vi "DAQ PID.vi"() -> ()   [LabVIEW 2024]
uses:
  <vilib>/addons/control/pid/pid.llb/PID (DBL).vi
  <vilib>/addons/control/pid/NI_PID_pid.lvlib
panel:
  out "2":bool
  out "1":bool
  out "ANG ACT":dbl
  out "error":dbl
  in  "stop":bool
  out "DERECHA":dbl
  out "IZQUIERDA":dbl
  out "P-A":dbl
  out "P-B":dbl
  out "DER":bool
  out "IZQ":bool
  out "PULSOS TOTALES":dbl
  in  "ANGULO":i16(knob) scale=-180.0..180.0
  in  "PID gains":T1 {"derivative time (Td, min)" format="%.3f"; "integral time (Ti, min)" format="%.3f"; "proportional gain (Kc)" format="%.3f"}
  out "ERROR":dbl(graph)
  out "PWM":dynamicdata(graph)
  out "SALIDA PID":dbl
  in  "output range":cluster{"output high":dbl, "output low":dbl} {"output low" format="%.2f"; "output high" format="%.2f"}
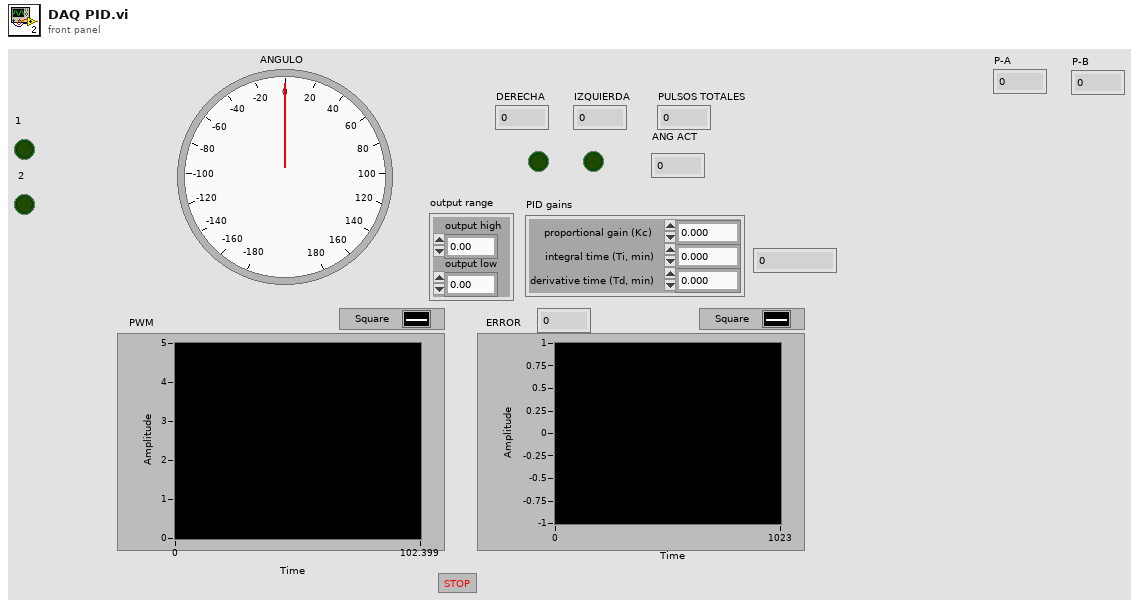
[diagram p1: front panel]
types:
  T1 = cluster{"proportional gain (Kc)":dbl, "integral time (Ti, min)":dbl, "derivative time (Td, min)":dbl}
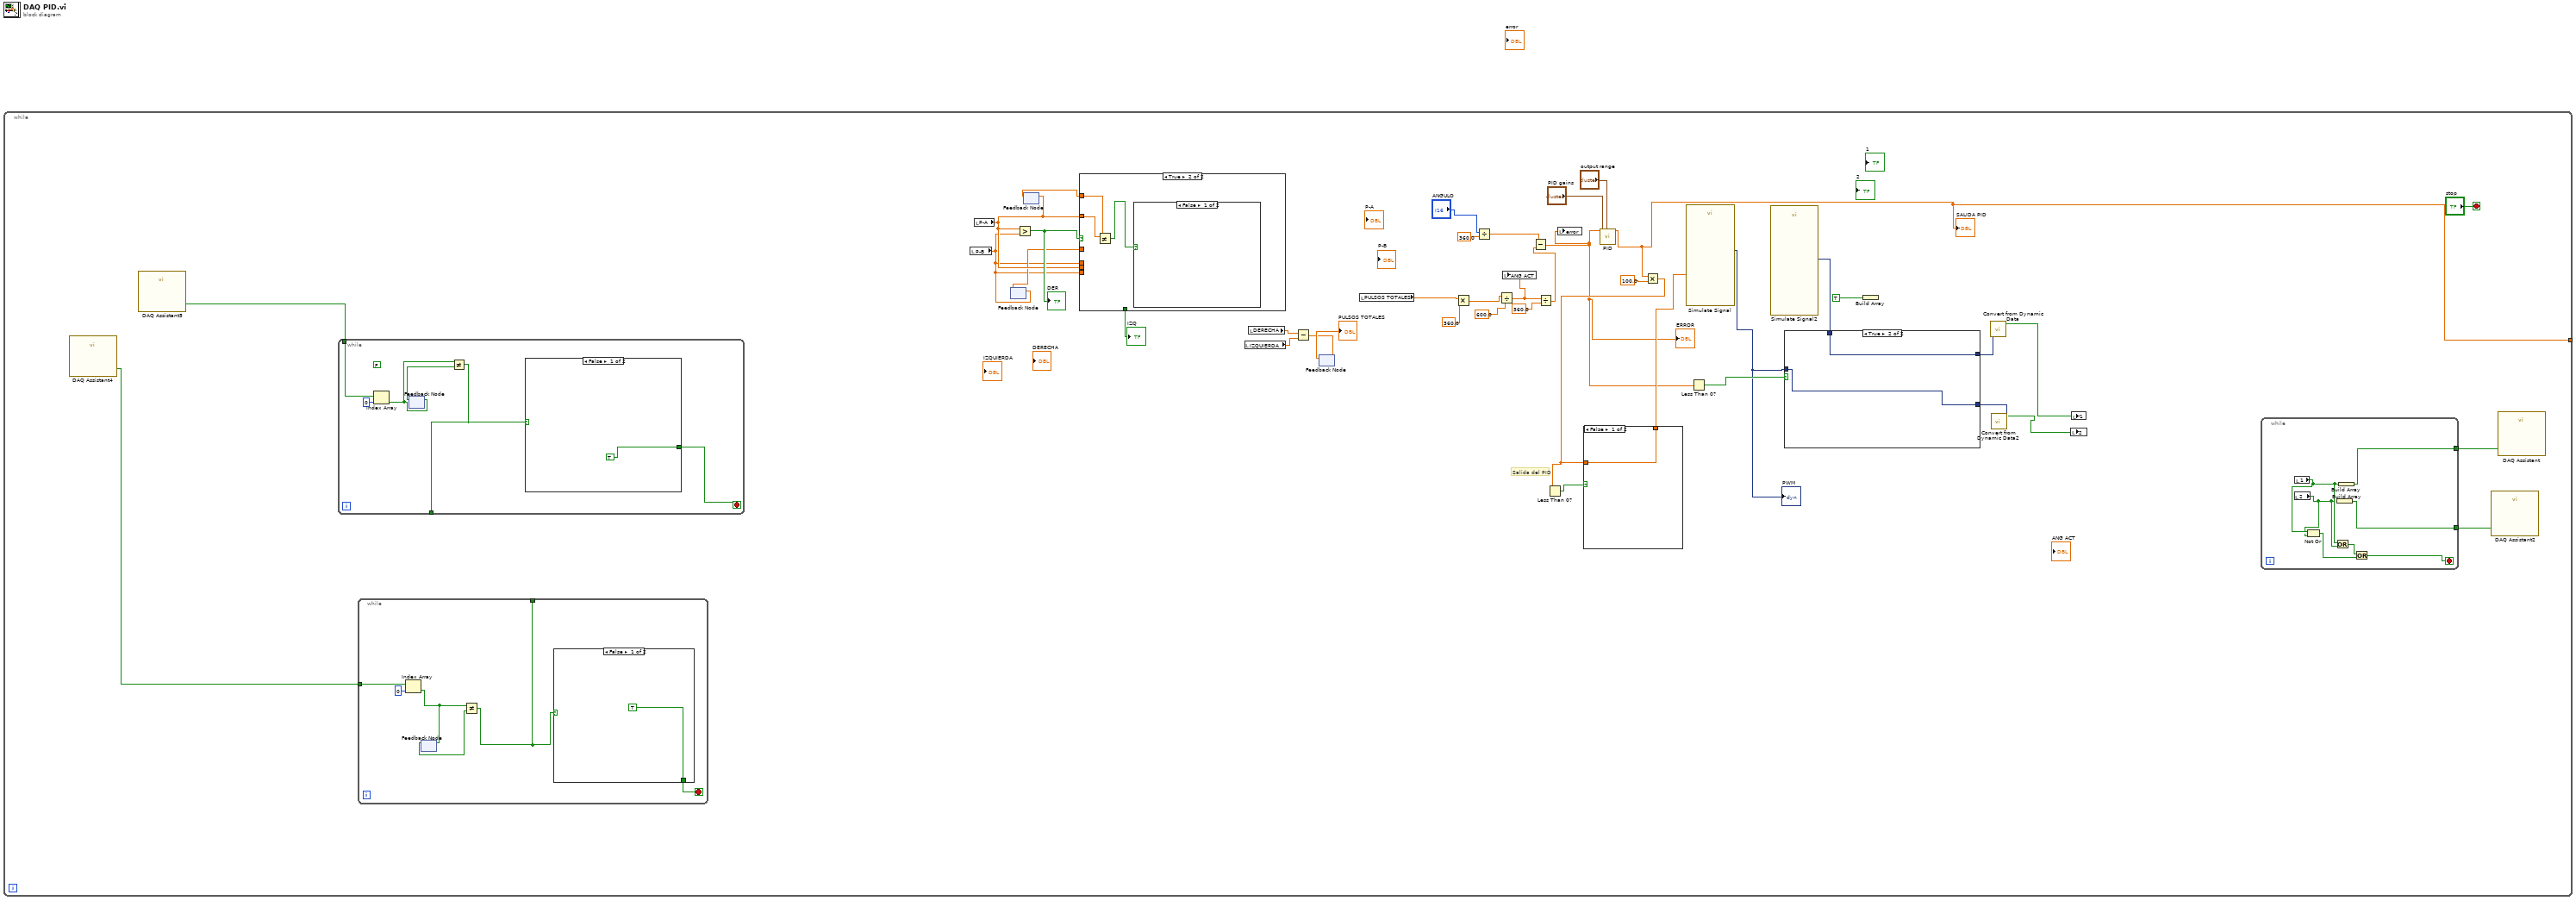
[diagram p0: block diagram]
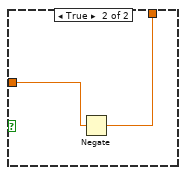
[diagram p2: hidden frame]
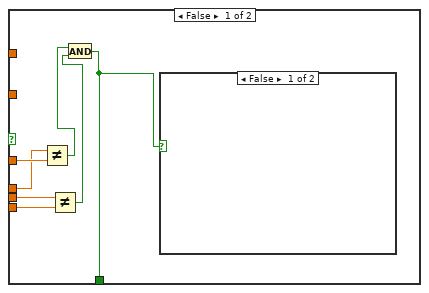
[diagram p4: hidden frame]
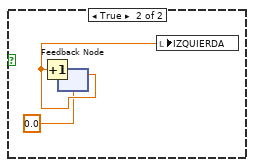
[diagram p5: hidden frame]
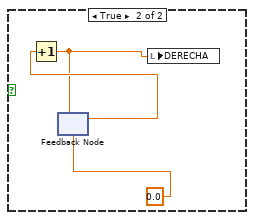
[diagram p6: hidden frame]
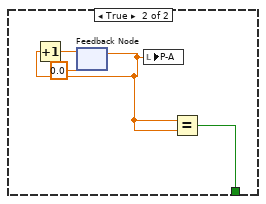
[diagram p7: hidden frame]
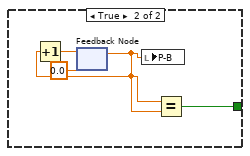
[diagram p8: hidden frame]
diagram:
  n1 = while {
    tunnel: [w3] -> _
    stop <- "stop" stop-if-true
    # "Salida del PID"
    n2 = call "DAQ Assistant4"() -> ("data"=w10:bool[])  [unwired: 17 in, 2 out]
    n3 = call "DAQ Assistant5"() -> ("data"=w9:bool[])  [unwired: 17 in, 2 out]
    n4 = while {
      tunnel: w9 -> [w85]
      tunnel: [w84] -> _
      stop <- w83 stop-if-true
      (unwired) FALSE
      n5 = Index Array(array=w85, index=0) -> (element=w87:bool)
      n6 = feedback #1() -> (w88:bool)  [unwired: 1 in]
      n7 = feedback-in #1(w87) -> ()
      n8 = Not Equal?(x=w87, y=w88) -> (x != y?=w84:bool)
      n9 = case shown="False" w84 {
        tunnel: [TRUE w90] -> w83
        frame False {
        }
        frame True {
          n10 = feedback #2(0.0) -> (w91:dbl)
          n11 = Increment(x=w91) -> (x+1=w93:dbl)
          n12 = feedback-in #2(w93) -> ()
          n13 = local write "P-B"(w91) -> ()
          n14 = Equal?(x=w91, y=w91) -> (x = y?=w90:bool)
        }
      }
    }
    n15 = while {
      tunnel: w10 -> [w74]
      tunnel: [w72] -> _
      stop <- w73 stop-if-true
      n16 = Index Array(array=w74, index=0) -> (element=w76:bool)
      n17 = feedback #3() -> (w77:bool)  [unwired: 1 in]
      n18 = feedback-in #3(w76) -> ()
      n19 = Not Equal?(x=w76, y=w77) -> (x != y?=w72:bool)
      n20 = case shown="False" w72 {
        tunnel: [TRUE w79] -> w73
        frame False {
        }
        frame True {
          n21 = feedback #4(0.0) -> (w80:dbl)
          n22 = Increment(x=w80) -> (x+1=w82:dbl)
          n23 = feedback-in #4(w82) -> ()
          n24 = local write "P-A"(w80) -> ()
          n25 = Equal?(x=w80, y=w80) -> (x = y?=w79:bool)
        }
      }
    }
    n26 = local read "P-B"() -> (w34:dbl)
    n27 = local read "P-A"() -> (w37:dbl)
    n28 = feedback #5() -> (w35:dbl)  [unwired: 1 in]
    n29 = feedback-in #5(w34) -> ()
    n30 = Greater?(x=w37, y=w34) -> (0:w40:bool)
    "DER" <- w40
    n31 = feedback #6() -> (w36:dbl)  [unwired: 1 in]
    n32 = feedback-in #6(w37) -> ()
    n33 = case shown="True" w40 {
      tunnel: w37 -> [w62 _]
      tunnel: w34 -> [w61 _]
      tunnel: w37 -> [_ w68]
      tunnel: w36 -> [_ w67]
      tunnel: w35 -> [w60 _]
      tunnel: w34 -> [w59 _]
      tunnel: [w56 _] -> w33
      frame False {
        n34 = Not Equal?(x=w59, y=w60) -> (x != y?=w57:bool)
        n35 = Not Equal?(x=w62, y=w61) -> (x != y?=w58:bool)
        n36 = And(x=w57, y=w58) -> (x .and. y?=w56:bool)
        n37 = case shown="False" w56 {
          frame False {
          }
          frame True {
            n38 = feedback #7(0.0) -> (w64:dbl)
            n39 = Increment(x=w64) -> (x+1=w65:dbl)
            n40 = feedback-in #7(w65) -> ()
            n41 = local write "IZQUIERDA"(w64) -> ()
          }
        }
      }
      frame True {
        n42 = Not Equal?(x=w68, y=w67) -> (x != y?=w66:bool)
        n43 = case shown="False" w66 {
          frame False {
          }
          frame True {
            n44 = feedback #8(0.0) -> (w71:dbl)
            n45 = Increment(x=w71) -> (x+1=w69:dbl)
            n46 = feedback-in #8(w69) -> ()
            n47 = local write "DERECHA"(w69) -> ()
          }
        }
      }
    }
    "IZQ" <- w33
    n48 = local read "IZQUIERDA"() -> (w38:dbl)
    n49 = local read "DERECHA"() -> (w39:dbl)
    n50 = Subtract(x=w39, y=w38) -> (x-y=w11:dbl)
    n51 = feedback #9() -> (→"PULSOS TOTALES":dbl)  [unwired: 1 in]
    n52 = feedback-in #9(w11) -> ()
    n53 = local read "PULSOS TOTALES"() -> (w28:dbl)
    n54 = Multiply(x=w28, y=360.0) -> (x*y=w27:dbl)
    n55 = Divide(x="ANGULO", y=360.0) -> (x/y=w29:dbl)
    n56 = Divide(x=w27, y=600.0) -> (x/y=w6:dbl)
    n57 = local write "ANG ACT"(w6) -> ()
    n58 = Divide(x=w6, y=360.0) -> (x/y=w7:dbl)
    n59 = Subtract(x=w29, y=w7) -> (x-y=w8:dbl)
    "ERROR" <- w8
    n60 = local write "error"(w8) -> ()
    n61 = call-poly <vilib>:"PID.vi"("output range"="output range", "PID gains"="PID gains", "setpoint"=w8) -> ("output"=w3:dbl)  [unwired: 7 in, 1 out]
    "SALIDA PID" <- w3
    n62 = Multiply(x=w3, y=100.0) -> (x*y=w19:dbl)
    n63 = Less Than 0?(x=w19) -> (x < 0?=w20:bool)
    n64 = case shown="False" w20 {
      tunnel: w19 -> [w49 w51]
      tunnel: [w49 w50] -> w18
      frame False {
      }
      frame True {
        n65 = Negate(x=w51) -> (-x=w50:dbl)
      }
    }
    n66 = call "Simulate Signal"("Duty Cycle (%)"=w18) -> ("Square"=w25:dynamicdata)  [unwired: 13 in, 1 out]
    "PWM" <- w25
    n67 = Less Than 0?(x=w8) -> (x < 0?=w26:bool)
    n68 = call "Simulate Signal2"() -> ("Square"=w23:dynamicdata)  [unwired: 14 in, 1 out]
    n69 = case shown="True" w26 {
      tunnel: w25 -> [w53 w54]
      tunnel: w23 -> [w52 w55]
      tunnel: [w53 w55] -> w22
      tunnel: [w52 w54] -> w21
      frame False {
      }
      frame True {
      }
    }
    n70 = Build Array(TRUE) -> ()  [unwired: 1 out]
    n71 = call "Convert from Dynamic Data"("Dynamic Data Type"=w22) -> ("Scalar"=w5:bool)  [unwired: 3 in]
    n72 = call "Convert from Dynamic Data2"("Dynamic Data Type"=w21) -> ("Scalar"=w4:bool)  [unwired: 3 in]
    n73 = local write "2"(w4) -> ()
    n74 = local write "1"(w5) -> ()
    n75 = while {
      tunnel: [w48] -> w2
      tunnel: [w47] -> w1
      stop <- w42 stop-if-true
      n76 = local read "2"() -> (w45:bool)
      n77 = local read "1"() -> (w46:bool)
      n78 = Not Or(1:w45, 2:w46) -> (0:w43:bool)
      n79 = Or(x=w46, y=w45) -> (x .or. y?=w44:bool)
      n80 = Build Array(w45) -> (w47:bool[])
      n81 = Build Array(w46) -> (w48:bool[])
      n82 = Or(x=w44, y=w43) -> (x .or. y?=w42:bool)
    }
    n83 = call "DAQ Assistant2"("data"=w1) -> ()  [unwired: 17 in, 2 out]
    n84 = call "DAQ Assistant"("data"=w2) -> ()  [unwired: 17 in, 2 out]
  }
